vi "OscillatorCtrlPan.vi"(8 "error in (no error)":errorcluster caption="entrée d'erreur (pas d'erreur)", 11 "EGG5210.lvclass":refnum<class "EGG5210.lvclass">) -> (0 "error out":errorcluster caption="sortie d'erreur", 3 "EGG5210.lvclass Out":refnum<class "EGG5210.lvclass">)   [LabVIEW 2010, in "EGG5210.lvclass"]
uses:
  EGG5210.lvclass
  BaseDevice/BaseDevice.lvclass
  <userlib>/EG_G 5210 LIA/ReadFunctions.ctl
panel:
  in  "Acq":bool
  in  "Ampl.(mV rms)":i32 min=0 max=5000 step=1
  in  "Freq. (Hz)":dbl
  in  "Stop":bool
  in  "MiseAJour":bool
  out "Init Program":bool
  # "EG&G 5210\nOscillator"
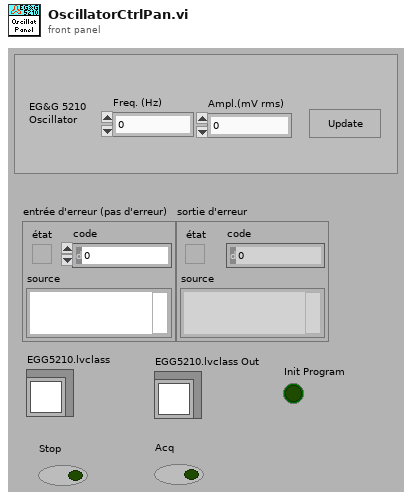
[diagram p1: front panel]
types:
  T1 = enum8{"Enabled", "Disabled", "Disabled and Grayed Out"}
  T2 = typedef "ReadFunctions.ctl" = enum16{"Sensitivity", "Vernier Mode", "Main Filter", "Filter Mode", "Line Filter", "Ref Source", "Ref Mode", "Ref Phase", "Ref Frequency", "Output Filter", "Time Constant", "Dyn Reserve", "X Offset", "Y Offset", "Expand Mode", "Int Oscillator", "Oscillator Freq", "All params", "Overload Byte", "Trigger Mode", "Error"}
  T3 = typedef "LockInPar.ctl" = cluster{"Sensitivity":u16, "Vernier Mode":bool, "Vernier Value":i32, "Main Filter":u16, "Filter Freq (Hz)":dbl, "Filter Mode":u16, " Line Notch":u16, "Reference":u16, "Reference Mode":u16, "Ref Phase (°)":dbl, "Ref Freq (Hz)":dbl, "Output Filter":u16, "Time Constant":u16, "Dynamic Res.":u16, "X Offset":bool, "X Offset Val %":dbl, "Y Offset":bool, "Y Offset Val %":dbl, "Expand":bool, "Osc Amp. (mV rms)":i32, "Int Osc (Hz)":dbl, "Trigger Mode":u16, "Input Mode":u16, "Ovld Source":u16}
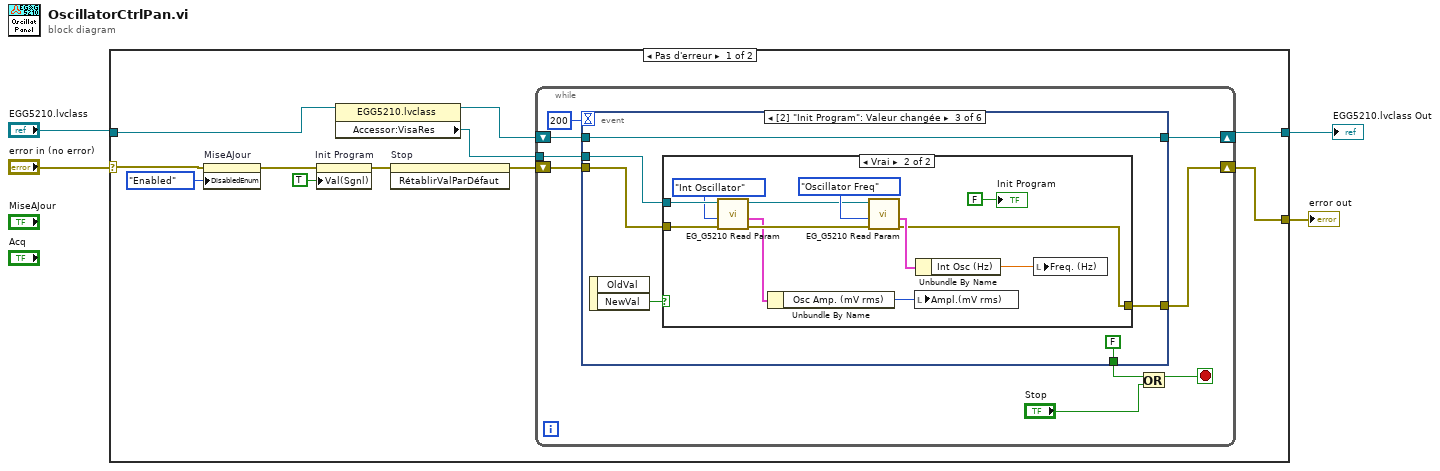
[diagram p0: block diagram]
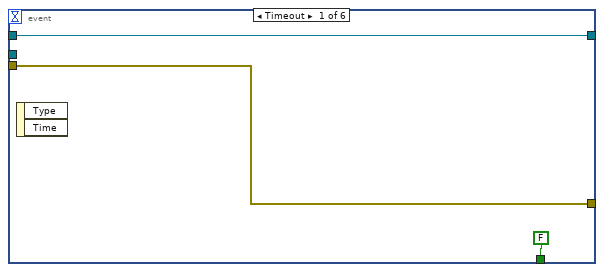
[diagram p2: hidden frame]
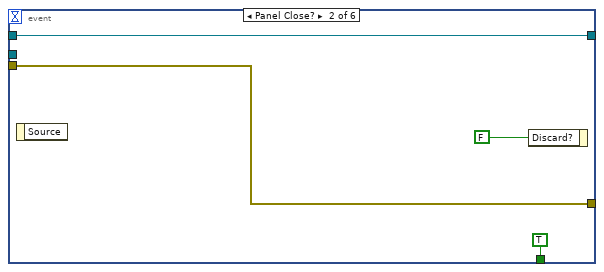
[diagram p3: hidden frame]
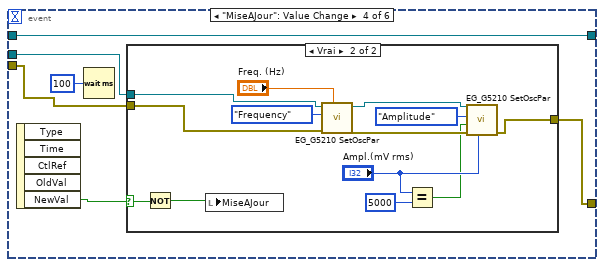
[diagram p5: hidden frame]
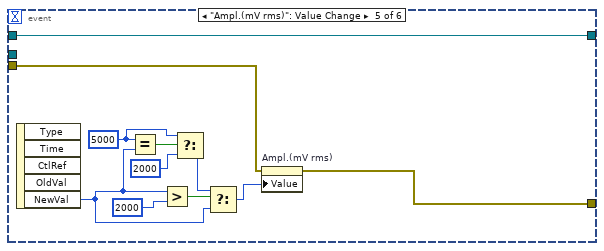
[diagram p7: hidden frame]
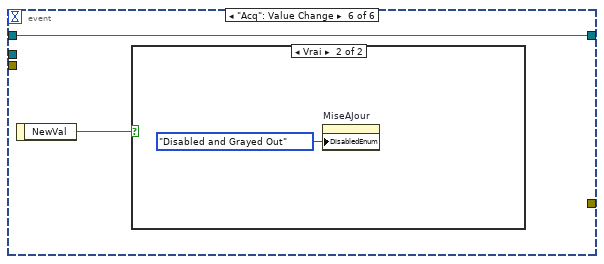
[diagram p8: hidden frame]
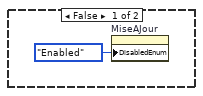
[diagram p9: hidden frame]
diagram:
  n1 = case shown="Pas d'erreur" "error in (no error)" {
    selector: "error in (no error)" -> [w6 w87]
    tunnel: [w15 w87] -> w3
    tunnel: "EGG5210.lvclass" -> [w10 w86]
    tunnel: [w13 w86] -> w2
    frame No Error {
      n2 = property on="MiseAJour" class="Bool (strict)"(error in=w6, "DisabledEnum"=T1."Enabled" ("Désactivé")) -> (error out=w5:errorcluster)  [unwired: 1 in, 1 out]
      n3 = property on="Init Program" class="Bool (strict)"(error in=w5, "Val(Sgnl)"=TRUE ("Valeur (Signalisation)")) -> (error out=w12:errorcluster)  [unwired: 1 in, 1 out]
      n4 = property class="EGG5210.lvclass"(reference=w10) -> (reference out=w9:refnum<class "EGG5210.lvclass">, "Accessor:VisaRes"=w8:refnum<visa-resource-name>)  [unwired: 1 in, 1 out]
      n5 = invoke on="Stop" class="Bool (strict)" method="RétablirValParDéfaut"(error in=w12) -> (error out=w11:errorcluster)  [unwired: 2 in, 2 out]
      n6 = while {
        shift-right: [w22] -> w15
        shift-left: w11 -> [w23]
        shift-right: [w19] -> w13
        shift-left: w9 -> [w21]
        tunnel: w8 -> [w16]
        stop <- w18 stop-if-true
        n7 = event shown="[2] \"Init Program\": Valeur changée" {
          selector: _ -> [_ _ _ _ _ _]
          dyn-events: _ -> [_ _ _ _ _ _]
          timeout: 200 -> [_ _ _ _ _ _]
          tunnel: w23 -> [w25 w29 w36 w52 w73 _]
          tunnel: [w25 w29 w35 w51 w72 _] -> w22
          tunnel: w21 -> [w26 w28 w34 w53 w71 w82]
          tunnel: [FALSE TRUE FALSE _ _ _] -> w20
          tunnel: [w26 w28 w34 w53 w71 w82] -> w19
          tunnel: w16 -> [_ _ w32 w54 _ _]
          event Timeout {
            n8 = event-data() -> ()  [unwired: 1 in, 2 out]
          }
          event Panel Close? {
            n9 = event-data() -> ()  [unwired: 1 in, 1 out]
            n10 = event-data("Discard?"=FALSE ("Rejeter ?")) -> ()  [unwired: 1 in, 1 out]
          }
          event "Init Program": Value Change {
            n11 = event-data() -> ("NewVal"=w37:bool)  [unwired: 1 in, 1 out]
            n12 = case shown="Vrai" w37 {
              tunnel: w36 -> [w38 w39]
              tunnel: [w38 w42] -> w35
              tunnel: w32 -> [_ w49]
              frame False {
              }
              frame True {
                n13 = call <userlib>:"EG_G5210 Read Param.vi"("error in (no error)"=w39, "Énum"=ReadFunctions."Int Oscillator", "Ressource VISA"=w49) -> ("error out"=w46:errorcluster, "LockInPar"=w44:T3, "Ressource VISA Out"=w45:refnum<visa-resource-name>)  [unwired: 5 in, 1 out]
                n14 = Unbundle By Name(w44) -> ("Osc Amp. (mV rms)"=w41:i32)
                n15 = call <userlib>:"EG_G5210 Read Param.vi"("error in (no error)"=w46, "Énum"=ReadFunctions."Oscillator Freq", "Ressource VISA"=w45) -> ("error out"=w42:errorcluster, "LockInPar"=w43:T3)  [unwired: 5 in, 2 out]
                n16 = local write "Ampl.(mV rms)"(w41) -> ()
                n17 = Unbundle By Name(w43) -> ("Int Osc (Hz)"=w40:dbl)
                n18 = local write "Freq. (Hz)"(w40) -> ()
                "Init Program" <- FALSE
              }
            }
          }
          event "MiseAJour": Value Change {
            n19 = event-data() -> ("NewVal"=w55:bool)  [unwired: 1 in, 4 out]
            n20 = Wait (ms)(milliseconds to wait=u32 100 ("attente (ms)")) -> ()  [unwired: 1 out]
            n21 = case shown="Vrai" w55 {
              selector: w55 -> [_ w70]
              tunnel: w54 -> [_ w65]
              tunnel: w52 -> [w57 w61]
              tunnel: [w57 w62] -> w51
              frame False {
              }
              frame True {
                n22 = Not(x=w70) -> (.not. x?=w69:bool)
                n23 = local write "MiseAJour"(w69) -> ()
                n24 = call <userlib>:"EG_G5210 SetOscPar.vi"("Frequency"="Freq. (Hz)", "error in (no error)"=w61, "Énum"=enum16{"Amplitude", "Frequency"}."Frequency", "Ressource VISA"=w65) -> ("error out"=w63:errorcluster, "Ressource VISA Out"=w64:refnum<visa-resource-name>)  [unwired: 6 in]
                n25 = Equal?(x="Ampl.(mV rms)", y=5000) -> (x = y?=w58:bool)
                n26 = call <userlib>:"EG_G5210 SetOscPar.vi"("Amplitude(mV rms)"="Ampl.(mV rms)", "error in (no error)"=w63, "Set to 5Vrms"=w58, "Énum"=enum16{"Amplitude", "Frequency"}."Amplitude", "Ressource VISA"=w64) -> ("error out"=w62:errorcluster)  [unwired: 5 in, 1 out]
              }
            }
          }
          event "Ampl.(mV rms)": Value Change {
            w76 = 5000 ("x")
            n27 = event-data() -> ("NewVal"=w78:i32)  [unwired: 1 in, 4 out]
            n28 = Equal?(x=w76, y=w78) -> (x = y?=w77:bool)
            n29 = Greater?(x=w78, y=2000) -> (0:w80:bool)
            n30 = Select(t=w76, s=w77, f=2000 ("y")) -> (s? t:f=w74:i32)
            n31 = Select(t=w74, s=w80, f=w78) -> (s? t:f=w79:i32)
            n32 = property on="Ampl.(mV rms)" class="NumDig (strict)"(error in=w73, "Value"=w79) -> (error out=w72:errorcluster)  [unwired: 1 in, 1 out]
          }
          event "Acq": Value Change {
            n33 = event-data() -> ("NewVal"=w83:bool)  [unwired: 1 in]
            n34 = case shown="Vrai" w83 {
              frame False {
                n35 = property on="MiseAJour" class="Bool (strict)"("DisabledEnum"=T1."Enabled" ("Désactivé")) -> ()  [unwired: 2 in, 2 out]
              }
              frame True {
                n36 = property on="MiseAJour" class="Bool (strict)"("DisabledEnum"=T1."Disabled and Grayed Out" ("Désactivé")) -> ()  [unwired: 2 in, 2 out]
              }
            }
          }
        }
        n37 = Or(x=w20, y="Stop") -> (x .or. y?=w18:bool)
      }
    }
    frame Error {
    }
  }
  "error out" <- w3
  "EGG5210.lvclass Out" <- w2
